vi "3D_Distance_FGV.vi"(8 "error in":errorcluster, 10 "FGV_Control":enum16{"Set", "Get"}(ring), 11 "3D in":T1) -> (0 "error out":errorcluster, 3 "3D out":T1)   [LabVIEW 2011]
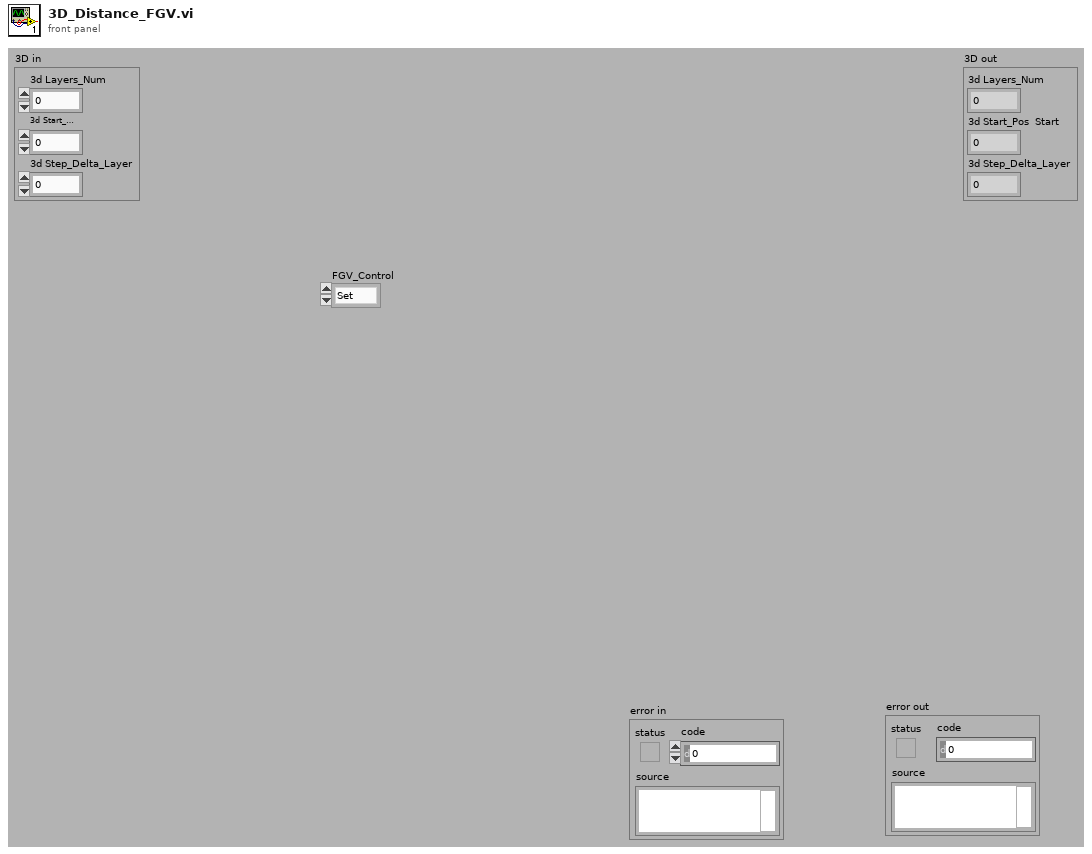
[diagram p1: front panel]
types:
  T1 = cluster{"3d Layers_Num":dbl, "3d Start_Pos  Start":dbl, "3d Step_Delta_Layer":dbl}
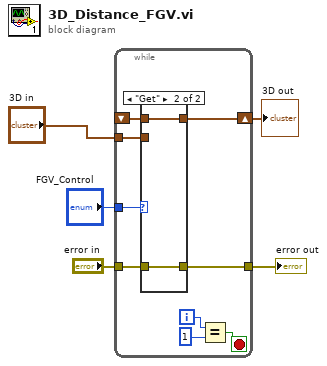
[diagram p0: block diagram]
diagram:
  n1 = while {
    tunnel: "3D in" -> [w14]
    shift-right: [w13] -> w1
    shift-left: _ -> [w12]
    tunnel: "error in" -> [w8]
    tunnel: [w7] -> w4
    tunnel: "FGV_Control" -> [w6]
    i -> [w9]
    stop <- w10 stop-if-true
    n2 = case shown="\"Get\"" w6 {
      tunnel: w14 -> [w16 _]
      tunnel: [w16 w18] -> w13
      tunnel: w12 -> [_ w18]
      tunnel: w8 -> [w15 w17]
      tunnel: [w15 w17] -> w7
      frame "Set", Default {
      }
      frame "Get" {
      }
    }
    n3 = Equal?(x=w9, y=1) -> (x = y?=w10:bool)
  }
  "error out" <- w4
  "3D out" <- w1
